vi "Test App Context of Nested App.vi"(8 "error in (no error)":errorcluster, 11 "Application Test in":refnum<class "Application Dev Test.lvclass">) -> (0 "error out":errorcluster, 3 "Application Test out":refnum<class "Application Dev Test.lvclass">)   [LabVIEW 2020, in "Application Dev Test.lvclass"]
uses:
  Application Dev Test.lvclass
  C:/Program Files (x86)/National Instruments/LabVIEW 2020/vi.lib/Astemes/LUnit/Test Case.lvclass
  source/Framework/Application/Application.lvclass
  C:/Git/astemes-triarc-framework/source/Framework/Process/Process.lvclass
  source/Framework/Process/Process.lvclass
  source/Framework/Process/Process.lvclass/Process.ctl
  source/Framework/Application/Application.lvclass/Application.ctl
  <vilib>/Astemes/LUnit/Test Case.lvclass/Test Case.ctl
  <vilib>/Astemes/LUnit/LUnit Assertion Result.lvclass/LUnit Assertion Result.ctl
  <vilib>/Astemes/LUnit/LUnit Test Case Result.lvclass/LUnit Test Case Result.ctl
  <vilib>/Astemes/LUnit/LUnit Method Result.lvclass/LUnit Method Result.ctl
  aa9c1303-abfb-423e-902a-0be9de222486.vi
  08d99f25-4927-4eee-98d7-9964e3a1bfe4.vi
  source/Framework/Application/Private/Add Process to Map.vi
  source/Framework/Application/Private/Start Idle Processes if Running.vi
  source/Framework/Application/Private/Throw Error If Process Already in App.vi
  source/Framework/Process/Protected/Messaging/Enqueue Message.vi
  source/Framework/Process/Public/Lifecycle/Get Lifecycle State.vi
  source/Framework/Process/Protected/SubVIs/Set Context.vi
  <vilib>/Astemes/LUnit/Palette/Pass.vi
  <vilib>/Astemes/LUnit/Palette/Fail.vi
  <vilib>/Astemes/LUnit/Compare Variants.vi
  <vilib>/Astemes/LUnit/Describe Comparison.vi
  <vilib>/Astemes/LUnit/Set Assertion Type.vi
  source/Framework/Process/Private/SubVIs/Wait for finish.vi
  source/Framework/Process/Private/SubVIs/Set Lifecycle State.vi
  source/Framework/Application/Public/Get Process.vi
  source/Framework/Process/Private/SubVIs/Handle Debug Data.vi
  <vilib>/Utility/error.llb/Clear Errors.vi
  source/Framework/Process/Public/Lifecycle/Leave Process Loop.vi
  <vilib>/Astemes/LUnit/Add test result.vi
  <vilib>/Astemes/LUnit/LUnit Write Passed.vi
  <vilib>/Astemes/LUnit/LUnit Write Message.vi
  <vilib>/Astemes/LUnit/LUnit Write Description.vi
  <vilib>/Astemes/LUnit/Variant to string.vi
  <vilib>/Astemes/LUnit/LUnit Write Assertion Type.vi
  source/Framework/Application/Private/Retrieve Process from App.vi
  source/Framework/Application/Private/Parse Process Name.vi
  source/Framework/Application/Private/Get Process from Map.vi
  source/Framework/Logging/Log Debug.vi
  <vilib>/AdvancedString/1D String Array to Delimited String.vi
  <vilib>/Utility/High Resolution Relative Seconds.vi
  <vilib>/Astemes/LUnit/LUnit Record Assertion Result.vi
  source/Framework/Process/Protected/Messaging/Request Message.vi
  <vilib>/AdvancedString/Delimited String to 1D String Array.vi
  <vilib>/Astemes/LUnit/LUnit Aggregate Assertion Results.vi
  source/Framework/Process/Private/SubVIs/Enqueue Request Message.vi
  <vilib>/Astemes/LUnit/Assertion Result/LUnit Read Status.vi
  <vilib>/Astemes/LUnit/LUnit Read Message.vi
  <vilib>/Astemes/LUnit/LUnit Read Description.vi
  <vilib>/Astemes/LUnit/Method Result/LUnit Merge Status.vi
  <vilib>/Astemes/LUnit/LUnit Concatenate result strings.vi
  <vilib>/Utility/error.llb/Error Cluster From Error Code.vi
  source/Framework/Process/Private/SubVIs/Wait for Response Message.vi
  <vilib>/Utility/Data Type/Get Type Information.vi
  <vilib>/Utility/LVClass/Get LV Class Name.vi
  <vilib>/Astemes/LUnit/LUnit Assertion Result.lvclass
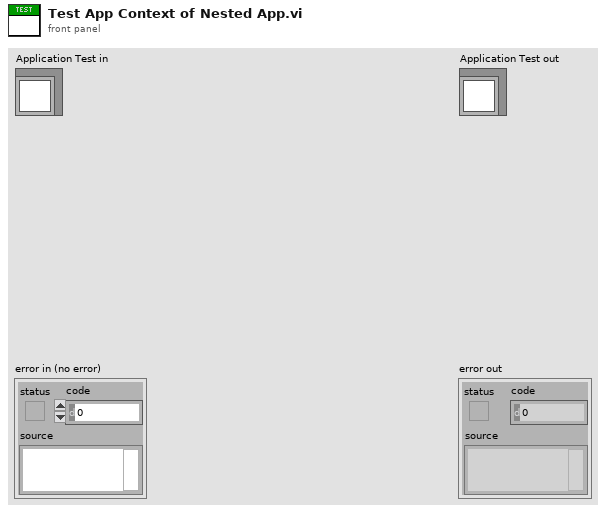
[diagram p1: front panel]
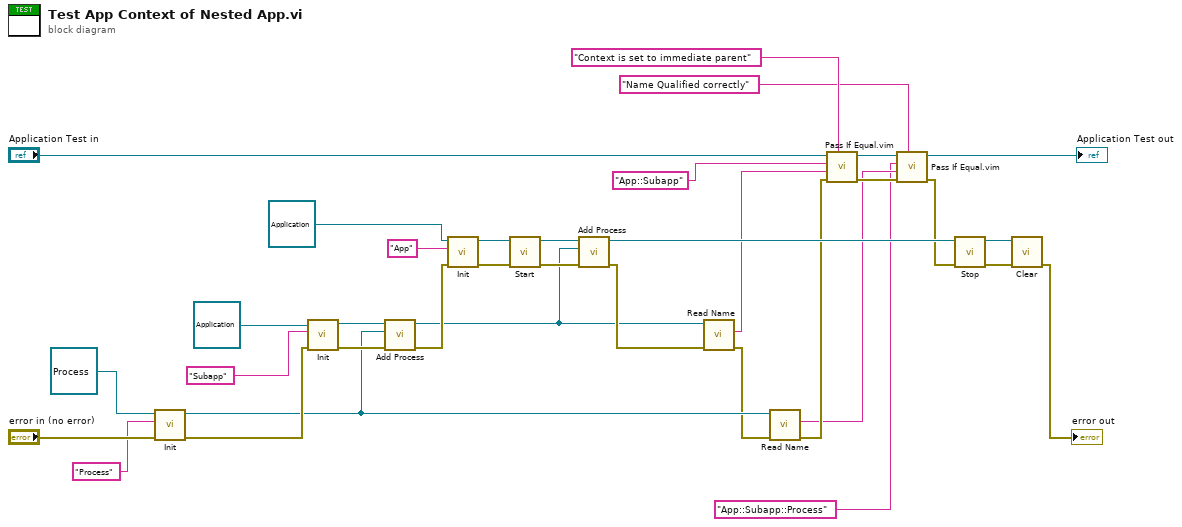
[diagram p0: block diagram]
diagram:
  n1 = call-dynamic "Init.vi"("error in (no error)"="error in (no error)", "Name"="Process", "Process In"=refnum<class "Process.lvclass"> refnum) -> ("error out"=w14:errorcluster, "Process Out"=w13:refnum<class "Process.lvclass">)  [unwired: 7 in]
  n2 = call-dynamic "Init.vi"("error in (no error)"=w14, "Name"="Subapp", "Process In"=refnum<class "Application.lvclass"> refnum ("Application.lvclass")) -> ("error out"=w19:errorcluster, "Process Out"=w20:refnum<class "Application.lvclass">)  [unwired: 7 in]
  n3 = call "Add Process.vi"("error in (no error)"=w19, "Process"=w13, "Application In"=w20) -> ("error out"=w18:errorcluster, "Application Out"=w1:refnum<class "Application.lvclass">)  [unwired: 7 in]
  n4 = call-dynamic "Init.vi"("error in (no error)"=w18, "Name"="App", "Process In"=refnum<class "Application.lvclass"> refnum ("Application.lvclass")) -> ("error out"=w34:errorcluster, "Process Out"=w35:refnum<class "Application.lvclass">)  [unwired: 7 in]
  n5 = call "Start.vi"("error in (no error)"=w34, "Process In"=w35) -> ("error out"=w32:errorcluster, "Process Out"=w22:refnum<class "Application.lvclass">)  [unwired: 7 in, 1 out]
  n6 = call "Add Process.vi"("error in (no error)"=w32, "Process"=w1, "Application In"=w22) -> ("error out"=w12:errorcluster, "Application Out"=w25:refnum<class "Application.lvclass">)  [unwired: 7 in]
  n7 = call "Read Name.vi"("error in (no error)"=w12, "Process In"=w1) -> ("error out"=w2:errorcluster, "Qualified Name"=w4:string)  [unwired: 6 in, 2 out]
  n8 = call "Read Name.vi"("error in (no error)"=w2, "Process In"=w13) -> ("error out"=w11:errorcluster, "Qualified Name"=w7:string)  [unwired: 6 in, 2 out]
  n9 = call "Pass If Equal.vim"("Description"="Context is set to immediate parent", "error in (no error)"=w11, "Actual"=w4, "Expected"="App::Subapp" ("Name"), "LUnit Test Case In"="Application Test in") -> ("error out"=w9:errorcluster, "LUnit Test Case Out"=w31:refnum<class "Application Dev Test.lvclass">)  [unwired: 5 in]
  n10 = call "Pass If Equal.vim"("Description"="Name Qualified correctly", "error in (no error)"=w9, "Actual"=w7, "Expected"="App::Subapp::Process" ("Name"), "LUnit Test Case In"=w31) -> ("error out"=w8:errorcluster, "LUnit Test Case Out"=→"Application Test out":refnum<class "Application Dev Test.lvclass">)  [unwired: 5 in]
  n11 = call "Stop.vi"("error in (no error)"=w8, "Process In"=w25) -> ("error out"=w28:errorcluster, "Process Out"=w33:refnum<class "Application.lvclass">)  [unwired: 7 in, 1 out]
  n12 = call-dynamic "Clear.vi"("error in (no error)"=w28, "Application In"=w33) -> ("error out"=→"error out":errorcluster)  [unwired: 9 in]
